vi "CheckWhileMotion.vi"(6 "Motor":i32=1, 8 "error In":errorcluster, 9 "Device Address In":i32, 10 "DeviceKey In":string, 11 "CmdLib In":refnum<k24>) -> (0 "error Out":errorcluster, 1 "Device Address Out":i32, 2 "DeviceKey Out":string, 3 "CmdLib Out":refnum<k24>, 5 "Is Motion Done":bool)   [LabVIEW 2013]
uses:
  C:/GEECS/Developers Version/source/Device Driver/Picomotor8742dotNet/NewFocus/CmdLib.dll
  CmdLib.dll
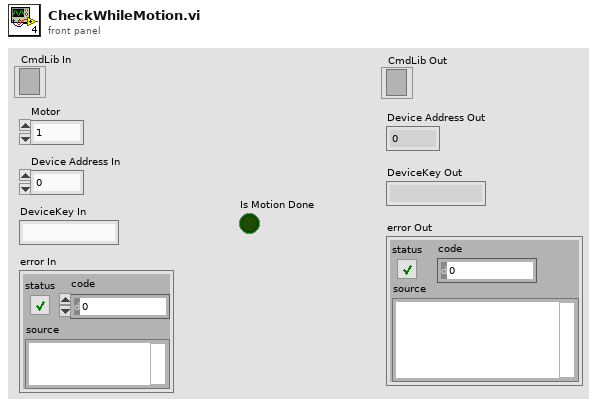
[diagram p1: front panel]
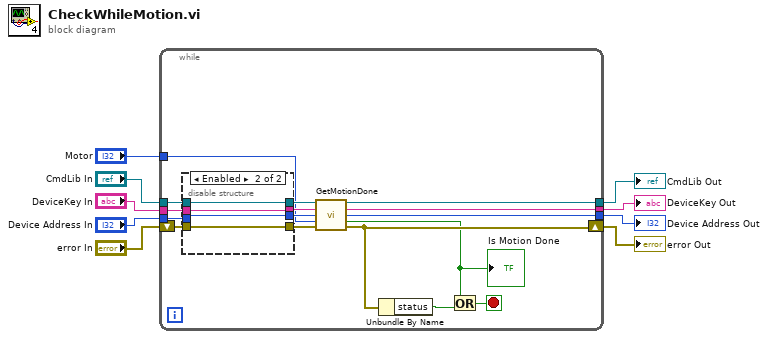
[diagram p0: block diagram]
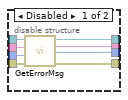
[diagram p2: hidden frame]
diagram:
  n1 = while {
    tunnel: "Motor" -> [w12]
    tunnel: "CmdLib In" -> [w23]
    tunnel: "DeviceKey In" -> [w22]
    tunnel: "Device Address In" -> [w19]
    shift-right: [w13] -> w2
    shift-left: "error In" -> [w21]
    tunnel: [w15] -> w4
    tunnel: [w16] -> w1
    tunnel: [w14] -> w3
    stop <- w17 stop-if-true
    n2 = disable-structure shown="Enabled" {
      disable-tunnel: [w33 w36] -> w25
      disable-tunnel: [w32 w37] -> w24
      disable-tunnel: w23 -> [w31 w37]
      disable-tunnel: w22 -> [w30 w36]
      disable-tunnel: w21 -> [w29 w34]
      disable-tunnel: [w28 w34] -> w20
      disable-tunnel: w19 -> [w27 w35]
      disable-tunnel: [w26 w35] -> w18
      frame Disabled {
        n3 = call "GetErrorMsg.vi"("error in (no error)"=w29, "Device Address In"=w27, "DeviceKey In"=w30, "CmdLib In"=w31) -> ("error out"=w28:errorcluster, "Device Address Out"=w26:i32, "DeviceKey Out"=w33:string, "CmdLib Out"=w32:refnum<k24>)
      }
      frame Enabled {
      }
    }
    n4 = call "GetMotionDone.vi"("CmdLib In"=w24, "DeviceKey In"=w25, "Device Address In"=w18, "Motor"=w12, "error in (no error)"=w20) -> ("CmdLib Out"=w16:refnum<k24>, "DeviceKey Out"=w15:string, "Device Address Out"=w14:i32, "Is Motion Done"=w11:bool, "error out"=w13:errorcluster)  [unwired: 6 in]
    "Is Motion Done" <- w11
    n5 = Unbundle By Name(w13) -> ("status"=w10:bool)
    n6 = Or(x=w11, y=w10) -> (x .or. y?=w17:bool)
  }
  "CmdLib Out" <- w1
  "DeviceKey Out" <- w4
  "Device Address Out" <- w3
  "error Out" <- w2
